vi "check_path_bin_file.vi"(8 "error in (no error)":errorcluster, 10 "Queue in":refnum<queue>, 11 "Files to transfer BIN in":path) -> (0 "error out":errorcluster, 2 "Queue out":refnum<queue>, 3 "Files to transfer BIN refnum out":refnum<file>)   [LabVIEW 2017, in "labview-standard-library.lvlib" / "file-transfer.lvlib"]
uses:
  file-transfer.lvlib
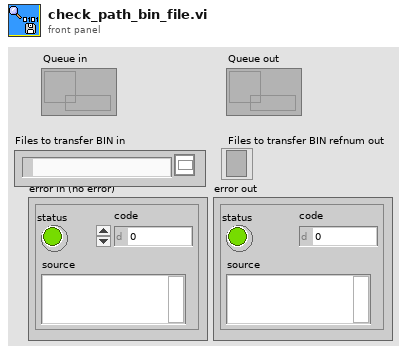
[diagram p1: front panel]
types:
  T1 = enum16{"open", "replace", "create", "open or create", "replace or create", "replace or create with confirmation"}
  T2 = enum16{"big-endian, network order", "native, host order", "little-endian"}
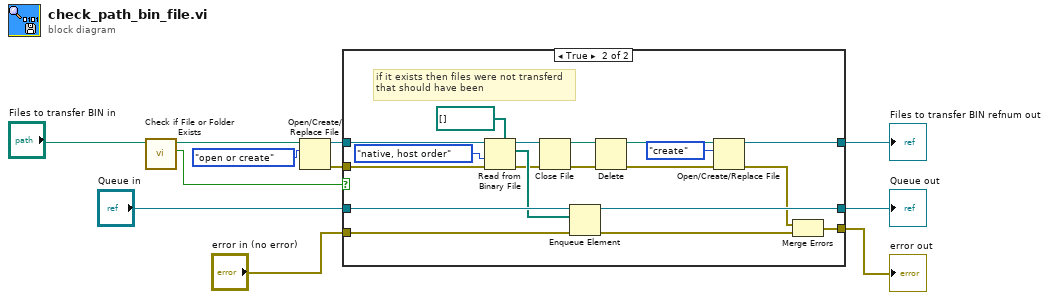
[diagram p0: block diagram]
diagram:
  n1 = call <vilib>:"Check if File or Folder Exists.vi"("path"="Files to transfer BIN in") -> ("file or folder exists?"=w8:bool, "dup path"=w1:path)  [unwired: 8 in, 1 out]
  n2 = Open/Create/Replace File(file path (use dialog)=w1, operation (0:open)=T1."open or create") -> (refnum out=w10:refnum<file>, error out=w9:errorcluster)  [unwired: 4 in, 1 out]
  n3 = case shown="True" w8 {
    tunnel: "Queue in" -> [w13 w33]
    tunnel: [w13 w32] -> w5
    tunnel: "error in (no error)" -> [w12 w31]
    tunnel: [w12 w16] -> w7
    tunnel: w9 -> [_ w29]
    tunnel: w10 -> [w14 w28]
    tunnel: [w14 w17] -> w11
    frame False {
      # "If it didn't exist and was just created\nno files were left over"
    }
    frame True {
      # "if it exists then files were not transferd\nthat should have been"
      n4 = Read from Binary File(5:path[] [], 8:w29, 9:T2."native, host order" ("byte order (0:big-endian, network order)"), 11:w28) -> (0:w23:errorcluster, 2:w26:path[], 3:w24:refnum<file>)  [unwired: 2 in, 1 out]
      n5 = Close File(refnum=w24, error in=w23) -> (path=w22:path, error out=w21:errorcluster)
      n6 = Enqueue Element(queue=w33, element=w26, error in (no error)=w31) -> (queue out=w32:refnum<queue>, error out=w30:errorcluster)  [unwired: 1 in, 1 out]
      n7 = Delete(path (use dialog)=w22, error in=w21) -> (deleted path=w19:path, error out=w20:errorcluster)  [unwired: 3 in, 1 out]
      n8 = Open/Create/Replace File(file path (use dialog)=w19, error in=w20, operation (0:open)=T1."create") -> (refnum out=w17:refnum<file>, error out=w15:errorcluster)  [unwired: 3 in, 1 out]
      n9 = Merge Errors(w15, w30) -> (w16:errorcluster)
    }
  }
  "Files to transfer BIN refnum out" <- w11
  "error out" <- w7
  "Queue out" <- w5
